vi "To String.vi"(8 "error in (no error)":errorcluster, 11 "Type Serializer in":refnum<class "Type Serializer.lvclass">) -> (0 "error out":errorcluster, 2 "String":string, 3 "Type Serializer out":refnum<class "Type Serializer.lvclass">)   [LabVIEW 2020, in "Protobuf RAW.lvlib" / "Type Serializer.lvclass"]
uses:
  Type Serializer.lvclass
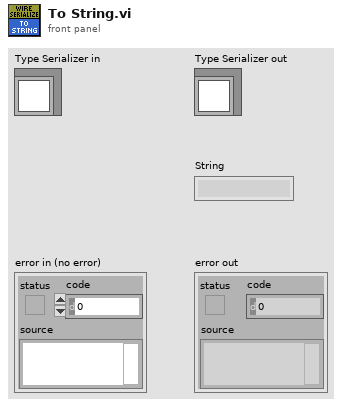
[diagram p1: front panel]
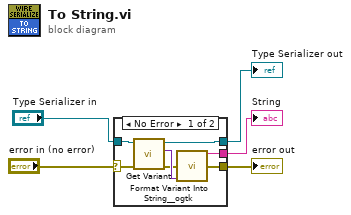
[diagram p0: block diagram]
diagram:
  n1 = case shown="No Error" "error in (no error)" {
    selector: "error in (no error)" -> [w8 w14]
    tunnel: [w7 w14] -> w4
    tunnel: [w9 w13] -> w2
    tunnel: "Type Serializer in" -> [w10 w13]
    tunnel: [w6 _] -> w1
    frame No Error {
      n2 = call-dynamic "Get Variant.vi"("error in (no error)"=w8, "Type Serializer in"=w10) -> ("error out"=w11:errorcluster, "Variant"=w12:variant, "Type Serializer out"=w9:refnum<class "Type Serializer.lvclass">)  [unwired: 7 in]
      n3 = call <userlib>:"Format Variant Into String__ogtk.vi"("error in (no error)"=w11, "Variant"=w12) -> ("Output String"=w6:string, "error out"=w7:errorcluster)  [unwired: 12 in]
    }
    frame Error {
    }
  }
  "error out" <- w4
  "Type Serializer out" <- w2
  "String" <- w1
